vi "Close Connection.vi"(8 "error in (no error)":errorcluster, 11 "HostDB in":refnum<class "SQLite.lvclass">) -> (0 "error out":errorcluster, 3 "HostDB out":refnum<class "SQLite.lvclass">)   [LabVIEW 2021, in "SQLite.lvclass"]
uses:
  SQLite.lvclass
  <vilib>/drjdpowell/SQLite Library/SQL Connection/Connection.lvclass
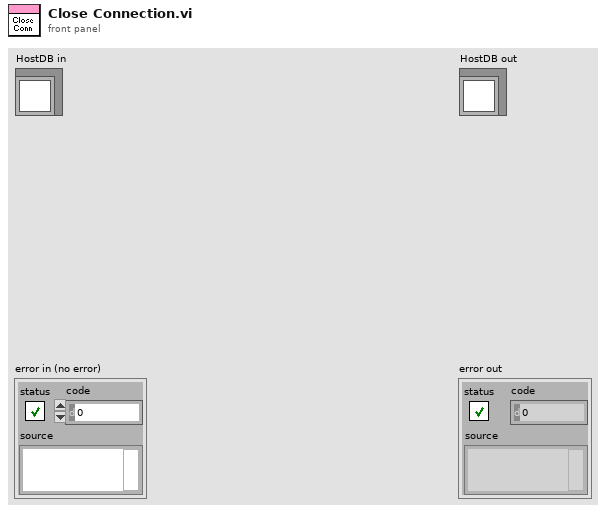
[diagram p1: front panel]
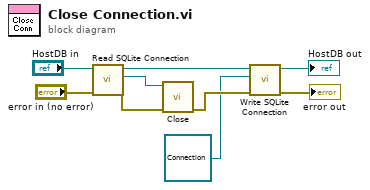
[diagram p0: block diagram]
diagram:
  n1 = call-dynamic "Read SQLite Connection.vi"("error in (no error)"="error in (no error)", "SQLite in"="HostDB in") -> ("error out"=w5:errorcluster, "SQLite.lvlib:Connection"=w8:refnum<class "Connection.lvclass">, "SQLite out"=w7:refnum<class "SQLite.lvclass">)  [unwired: 7 in]
  n2 = call-dynamic "Close.vi"("error in (no error)"=w5, "SQLite Connection in"=w8) -> ("error out"=w4:errorcluster)  [unwired: 9 in]
  n3 = call-dynamic "Write SQLite Connection.vi"("error in (no error)"=w4, "SQLite.lvlib:Connection"=refnum<class "Connection.lvclass"> refnum, "SQLite in"=w7) -> ("error out"=→"error out":errorcluster, "SQLite out"=→"HostDB out":refnum<class "SQLite.lvclass">)  [unwired: 7 in]
